vi "ad get line direction.vi"(8 "error in (no error)":errorcluster, 9 "mask":u32, 10 "cha":i32, 11 "adh":i32) -> (0 "error out":errorcluster, 1 "mask out":u32, 3 "function return":i32)   [LabVIEW 2021, in "libad4.lvlib"]
doc: "LIBAD4 function: ad_get_line_direction (int32_t adh, int32_t cha, uint32_t *mask);\n\nReturns the direction of the digital lines."
uses:
  <userlib>/libad4/libad4.lvlib
  <userlib>/libad4/libad4.dll
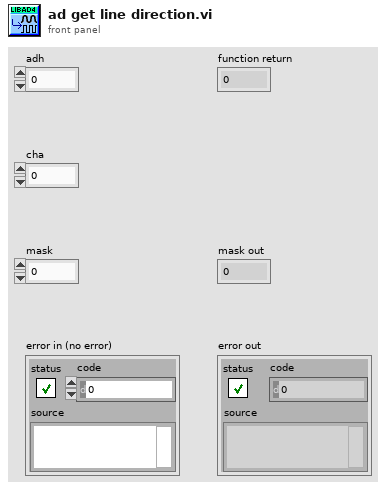
[diagram p1: front panel]
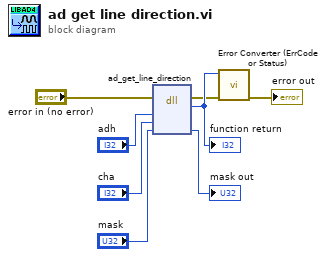
[diagram p0: block diagram]
diagram:
  n1 = dll-call lib="C:/Program Files/National Instruments/LabVIEW 2021/user.lib/libad4/libad4.*" fn="ad_get_line_direction"(error in="error in (no error)", "adh"="adh", "cha"="cha", "mask"="mask") -> (error out=w2:errorcluster, w8:i32, "mask"=→"mask out":u32)  [unwired: 4 in, 1 out]
  "function return" <- w8
  n2 = call <userlib>:"Error Converter (ErrCode or Status).vi"("error in (no error)"=w2, "error code"=w8) -> ("error out"=→"error out":errorcluster)  [unwired: 9 in]
